vi "TrendsD26.vi"() -> ()   [LabVIEW 2019, in "D01.lvlib"]
uses:
  D01.lvlib
panel:
  out "No Change":bool
  out "Sudden Change":bool
  out "Decrease":bool
  out "Increase":bool
  out "Previous  ES":dbl
  out "Present  Speed":dbl
  out "Present Error":dbl format="%#.2g"
  out "Previous Error":dbl
  out "Previous  Speed":dbl
  out "Previous PW":dbl caption="Control Information"
  out "Pulse Trends":waveform(i16)[](graph) caption="Waveform Chart - Dark"
  in  "Close":bool
  out "disc name":string="Disc 01 Trends"
  out "dsgs":string="DSGS"
  out "Speed Trend":waveform(dbl)(graph) caption="Waveform Chart - Dark"
  out "Average Trend":waveform(dbl)[](graph) caption="Waveform Chart - Dark"
  out "Live Trend":waveform(dbl)[](graph) caption="Waveform Chart - Dark"
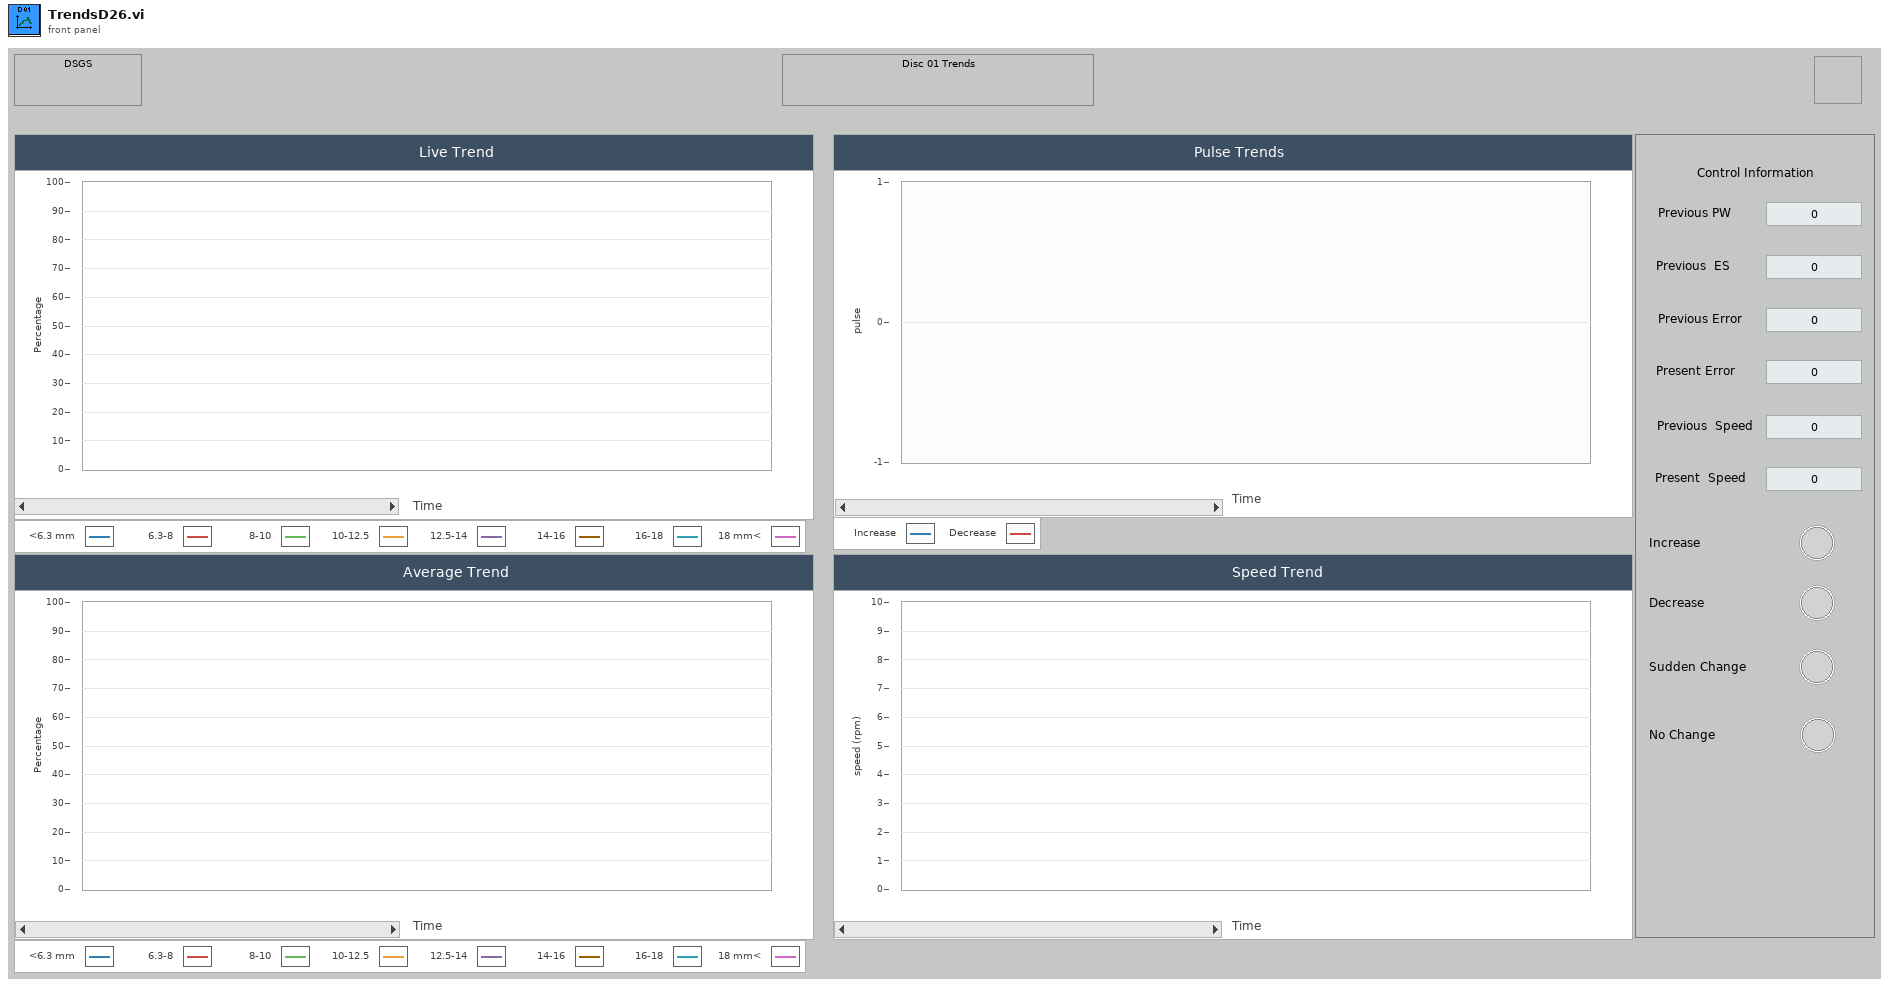
[diagram p1: front panel]
types:
  T1 = cluster{"decrease D26":bool, "increase D26":bool, "no change D26":bool, "sudden change D26":bool, "last error 26":dbl, "previous speed D26":dbl, "puls width D26":dbl, "slope D26":dbl}
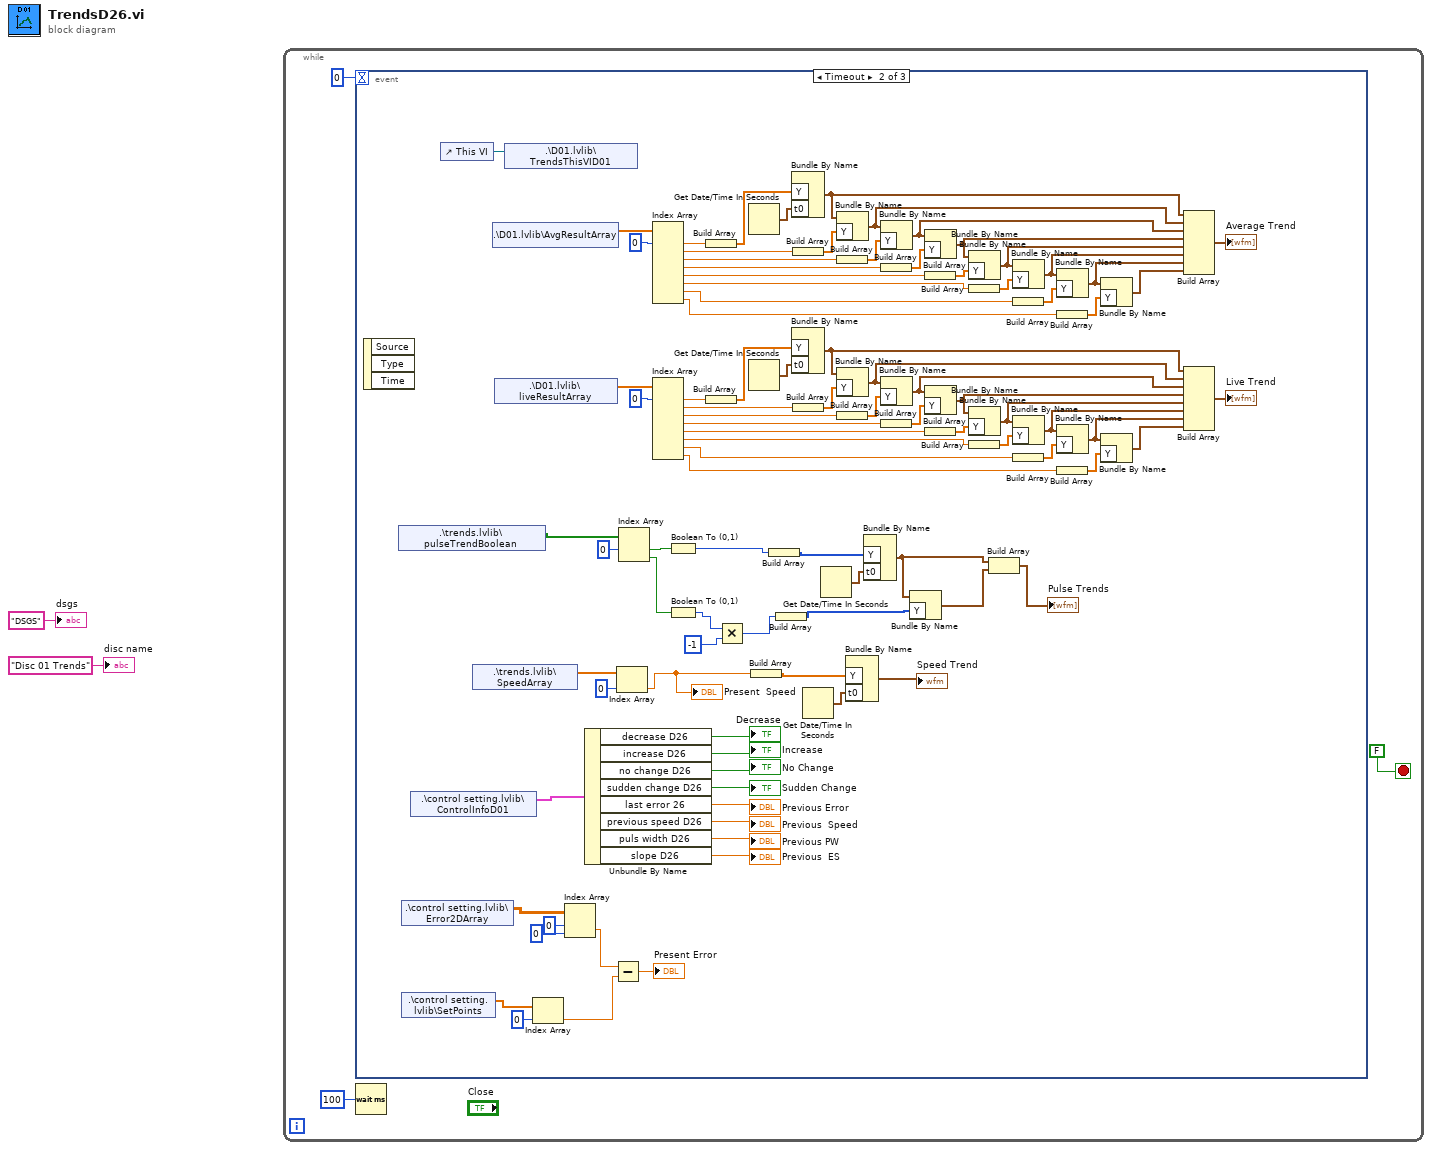
[diagram p0: block diagram]
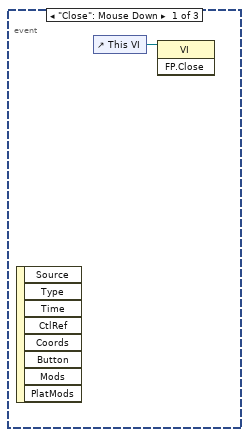
[diagram p2: hidden frame]
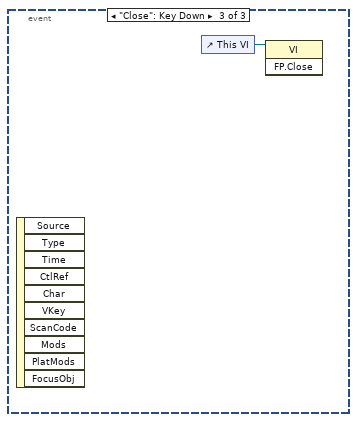
[diagram p3: hidden frame]
diagram:
  n1 = while {
    stop <- FALSE stop-if-true
    n2 = event shown="[1] Timeout" {
      selector: _ -> [_ _ _]
      dyn-events: _ -> [_ _ _]
      timeout: 0 -> [_ _ _]
      event "Close": Mouse Down {
        n3 = event-data() -> ()  [unwired: 1 in, 8 out]
        n4 = control-ref of="This VI"() -> (w6:refnum<vi>)
        n5 = invoke class="VI" method="FP.Close"(reference=w6) -> ()  [unwired: 2 in, 3 out]
      }
      event Timeout {
        n6 = event-data() -> ()  [unwired: 1 in, 3 out]
        n7 = shared-variable ".\\trends.lvlib\\pulseTrendBoolean"() -> (w40:bool[])  [unwired: 1 in, 1 out]
        n8 = shared-variable ".\\control setting.lvlib\\Error2DArray"() -> (w18:dbl[][])  [unwired: 1 in, 1 out]
        n9 = shared-variable ".\\control setting.lvlib\\SetPoints"() -> (w11:dbl[])  [unwired: 1 in, 1 out]
        n10 = shared-variable ".\\control setting.lvlib\\ControlInfoD01"() -> (w24:T1)  [unwired: 1 in, 1 out]
        n11 = control-ref of="This VI"() -> (w44:refnum<vi>)
        n12 = shared-variable ".\\trends.lvlib\\SpeedArray"() -> (w29:dbl[])  [unwired: 1 in, 1 out]
        n13 = shared-variable ".\\D01.lvlib\\AvgResultArray"() -> (w53:dbl[])  [unwired: 1 in, 1 out]
        n14 = shared-variable ".\\D01.lvlib\\liveResultArray"() -> (w100:dbl[])  [unwired: 1 in, 1 out]
        n15 = shared-variable ".\\D01.lvlib\\TrendsThisVID01"(w44) -> ()  [unwired: 1 in, 1 out]
        n16 = Index Array(array=w11, index=0) -> (element=w8:dbl)
        n17 = Index Array(array=w18, index (row)=0, index (col)=0 ("disabled index (col)")) -> (element=w9:dbl)
        n18 = Unbundle By Name(w24) -> ("decrease D26"=→"Decrease":bool, "increase D26"=→"Increase":bool, "no change D26"=→"No Change":bool, "sudden change D26"=→"Sudden Change":bool, "last error 26"=→"Previous Error":dbl, "previous speed D26"=→"Previous  Speed":dbl, "puls width D26"=→"Previous PW":dbl, "slope D26"=→"Previous  ES":dbl)
        n19 = Subtract(x=w9, y=w8) -> (x-y=→"Present Error":dbl)
        n20 = Index Array(array=w29, index=0) -> (element=w15:dbl)
        "Present  Speed" <- w15
        n21 = Index Array(array=w40, index #1=0 ("index")) -> (element #1=w39:bool, element #2=w37:bool)  [unwired: 1 in]
        n22 = Index Array(array=w53, index #1=0 ("index")) -> (element #1=w64:dbl, element #2=w65:dbl, element #3=w67:dbl, element #4=w69:dbl, element #5=w70:dbl, element #6=w72:dbl, element #7=w74:dbl, element #8=w49:dbl)  [unwired: 7 in]
        n23 = Index Array(array=w100, index #1=0 ("index")) -> (element #1=w89:dbl, element #2=w88:dbl, element #3=w86:dbl, element #4=w84:dbl, element #5=w83:dbl, element #6=w81:dbl, element #7=w79:dbl, element #8=w45:dbl)  [unwired: 7 in]
        n24 = Boolean To (0,1)(Boolean=w39) -> (0, 1=w38:i16)
        n25 = Boolean To (0,1)(Boolean=w37) -> (0, 1=w33:i16)
        n26 = Build Array(w64) -> (w75:dbl[])
        n27 = Build Array(w89) -> (w78:dbl[])
        n28 = Multiply(x=w33, y=i16 -1 ("0, 1")) -> (x*y=w31:i16)
        n29 = Get Date/Time In Seconds() -> (seconds since 1Jan1904=w57:timestamp)
        n30 = Get Date/Time In Seconds() -> (seconds since 1Jan1904=w97:timestamp)
        n31 = Build Array(w15) -> (w27:dbl[])
        n32 = Build Array(w38) -> (w41:i16[])
        n33 = Build Array(w31) -> (w36:i16[])
        n34 = Bundle By Name("Y"=w75, "t0"=w57) -> (w63:waveform(dbl))  [unwired: 1 in]
        n35 = Bundle By Name("Y"=w78, "t0"=w97) -> (w91:waveform(dbl))  [unwired: 1 in]
        n36 = Build Array(w65) -> (w66:dbl[])
        n37 = Build Array(w88) -> (w87:dbl[])
        n38 = Get Date/Time In Seconds() -> (seconds since 1Jan1904=w26:timestamp)
        n39 = Get Date/Time In Seconds() -> (seconds since 1Jan1904=w42:timestamp)
        n40 = Bundle By Name(cluster=w63, "Y"=w66) -> (w62:waveform(dbl))
        n41 = Build Array(w67) -> (w68:dbl[])
        n42 = Bundle By Name(cluster=w91, "Y"=w87) -> (w92:waveform(dbl))
        n43 = Build Array(w86) -> (w85:dbl[])
        n44 = Bundle By Name("Y"=w27, "t0"=w26) -> (→"Speed Trend":waveform(dbl))  [unwired: 1 in]
        n45 = Bundle By Name("Y"=w41, "t0"=w42) -> (w35:waveform(i16))  [unwired: 1 in]
        n46 = Bundle By Name(cluster=w62, "Y"=w68) -> (w61:waveform(dbl))
        n47 = Build Array(w69) -> (w56:dbl[])
        n48 = Bundle By Name(cluster=w92, "Y"=w85) -> (w93:waveform(dbl))
        n49 = Build Array(w84) -> (w98:dbl[])
        n50 = Bundle By Name(cluster=w35, "Y"=w36) -> (w34:waveform(i16))
        n51 = Bundle By Name(cluster=w61, "Y"=w56) -> (w60:waveform(dbl))
        n52 = Build Array(w70) -> (w71:dbl[])
        n53 = Bundle By Name(cluster=w93, "Y"=w98) -> (w94:waveform(dbl))
        n54 = Build Array(w83) -> (w82:dbl[])
        n55 = Bundle By Name(cluster=w60, "Y"=w71) -> (w59:waveform(dbl))
        n56 = Build Array(w72) -> (w73:dbl[])
        n57 = Bundle By Name(cluster=w94, "Y"=w82) -> (w95:waveform(dbl))
        n58 = Build Array(w81) -> (w80:dbl[])
        n59 = Build Array(w35, w34) -> (→"Pulse Trends":waveform(i16)[])
        n60 = Bundle By Name(cluster=w59, "Y"=w73) -> (w58:waveform(dbl))
        n61 = Build Array(w74) -> (w76:dbl[])
        n62 = Bundle By Name(cluster=w95, "Y"=w80) -> (w96:waveform(dbl))
        n63 = Build Array(w79) -> (w77:dbl[])
        n64 = Bundle By Name(cluster=w58, "Y"=w76) -> (w51:waveform(dbl))
        n65 = Build Array(w49) -> (w52:dbl[])
        n66 = Bundle By Name(cluster=w96, "Y"=w77) -> (w46:waveform(dbl))
        n67 = Build Array(w45) -> (w48:dbl[])
        n68 = Bundle By Name(cluster=w51, "Y"=w52) -> (w50:waveform(dbl))
        n69 = Bundle By Name(cluster=w46, "Y"=w48) -> (w47:waveform(dbl))
        n70 = Build Array(w63, w62, w61, w60, w59, w58, w51, w50) -> (→"Average Trend":waveform(dbl)[])
        n71 = Build Array(w91, w92, w93, w94, w95, w96, w46, w47) -> (→"Live Trend":waveform(dbl)[])
      }
      event "Close": Key Down {
        n72 = event-data() -> ()  [unwired: 1 in, 10 out]
        n73 = control-ref of="This VI"() -> (w101:refnum<vi>)
        n74 = invoke class="VI" method="FP.Close"(reference=w101) -> ()  [unwired: 2 in, 3 out]
      }
    }
    n75 = Wait (ms)(milliseconds to wait=u32 100) -> ()  [unwired: 1 out]
  }
  "disc name" <- "Disc 01 Trends" ("disc name")
  "dsgs" <- "DSGS" ("dsgs")
